vi "Teleop.vi"(0 "Call Context":T3) -> (1 "Loop 5 Value 1":dbl, 2 "Loop 5 Value 2":dbl, 3 "Loop 2 Value 2":dbl, 4 "Loop 2 Value 1":dbl, 6 "Loop 0 Value 1":dbl, 7 "Loop 1 Value 2":dbl, 8 "Loop 4 Value 2":dbl, 9 "SubState 5":T1, 10 "Loop 0 Value 2":dbl, 11 "Loop 1 Value 1":dbl, 12 "Loop 3 Value 2":dbl, 13 "Loop 3 Value 1":dbl, 14 "SubState 0":T2=enum."driver control", 15 "SubState 4":T2, 16 "SubState 3":T2, 17 "SubState 1":T2, 18 "Loop 4 Value 1":dbl, 19 "SubState 2":T2)   [LabVIEW 2011]
uses:
  subStates.ctl
  <vilib>/Rock Robotics/WPI/DriverStation/WPI_DriverStationDerivedRobotMode.ctl
  singleUseSubstate.ctl
  fg_typedef.ctl
  <vilib>/Rock Robotics/WPI/Solenoid/WPI_SolenoidValue.ctl
  <vilib>/Rock Robotics/WPI/Solenoid/WPI_SolenoidGetEnum.vi
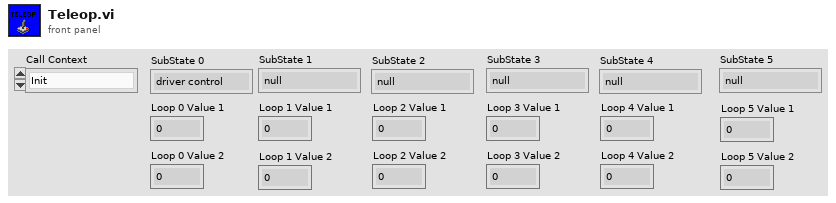
[diagram p1: front panel]
types:
  T1 = typedef "singleUseSubstate.ctl" = enum16{"null", "wait", "shift", "shift high", "shift low", "bridge down", "bridge up", "extender in", "extender out", "extender toggle", "end"}
  T2 = typedef "subStates.ctl" = enum16{"null", "wait", "driver control", "auto", "manual override", "autoDrive", "hold position", "rotate", "end"}
  T3 = typedef "WPI_DriverStationDerivedRobotMode.ctl" = enum16{"Init", "Execute", "Stop"}
  T4 = typedef "fg_typedef.ctl" = enum16{"Get", "Set"}
  T5 = typedef "WPI_JoystickDevRef.ctl" = cluster{"Device":T6}
  T6 = typedef "WPI_JoystickDeviceEnum.ctl" = enum16{"USB 1", "USB 2", "USB 3", "USB 4", "Kinect 1", "Kinect 2"}
  T7 = typedef "WPI_JoystickButtonState.ctl" = cluster{"Button 1":bool, "Button 2":bool, "Button 3":bool, "Button 4":bool, "Button 5":bool, "Button 6":bool, "Button 7":bool, "Button 8":bool, "Button 9":bool, "Button 10":bool, "Button 11":bool, "Button 12":bool}
  T8 = cluster{"axis 1 (x)":dbl, "axis 2 (y)":dbl, "axis 3 (throttle)":dbl, "axis 4":dbl, "axis 5":dbl, "axis 6":dbl}
  T9 = typedef "WPI_EncoderDevRef.ctl" = cluster{"DevStatus":errorcluster, "EncoderIndex":T10, "CounterIndex":T11, "DistancePerCount":dbl, "Decoding Type":T12}
  T10 = typedef "FPGA_EncoderIdx.ctl" = enum8{"Enc 0", "Enc 1", "Enc 2", "Enc 3", "Invalid"}
  T11 = typedef "FPGA_CounterCtrSystemIndex.ctl" = enum8{"Ctr 0", "Ctr 1", "Ctr 2", "Ctr 3", "Ctr 4", "Ctr 5", "Ctr 6", "Ctr 7", "Invalid"}
  T12 = typedef "WPI_EncoderType.ctl" = enum16{"1x", "2x", "4x"}
  T13 = typedef "WPI_SolenoidValue.ctl" = enum16{"Off", "On", "Forward", "Reverse"}
  T14 = typedef "WPI_SolenoidDevRef.ctl" = cluster{"DevStatus":errorcluster, "Solenoid Module":T15, "Forward Solenoid Channel":T16, "Reverse Solenoid Channel":T16}
  T15 = typedef "FPGA_TypedefSolenoidModule.ctl" = enum16{"Solenoid Module 1", "Solenoid Module 2"}
  T16 = typedef "WPI_SolenoidChannel.ctl" = enum8{"Solenoid 1", "Solenoid 2", "Solenoid 3", "Solenoid 4", "Solenoid 5", "Solenoid 6", "Solenoid 7", "Solenoid 8", "Invalid"}
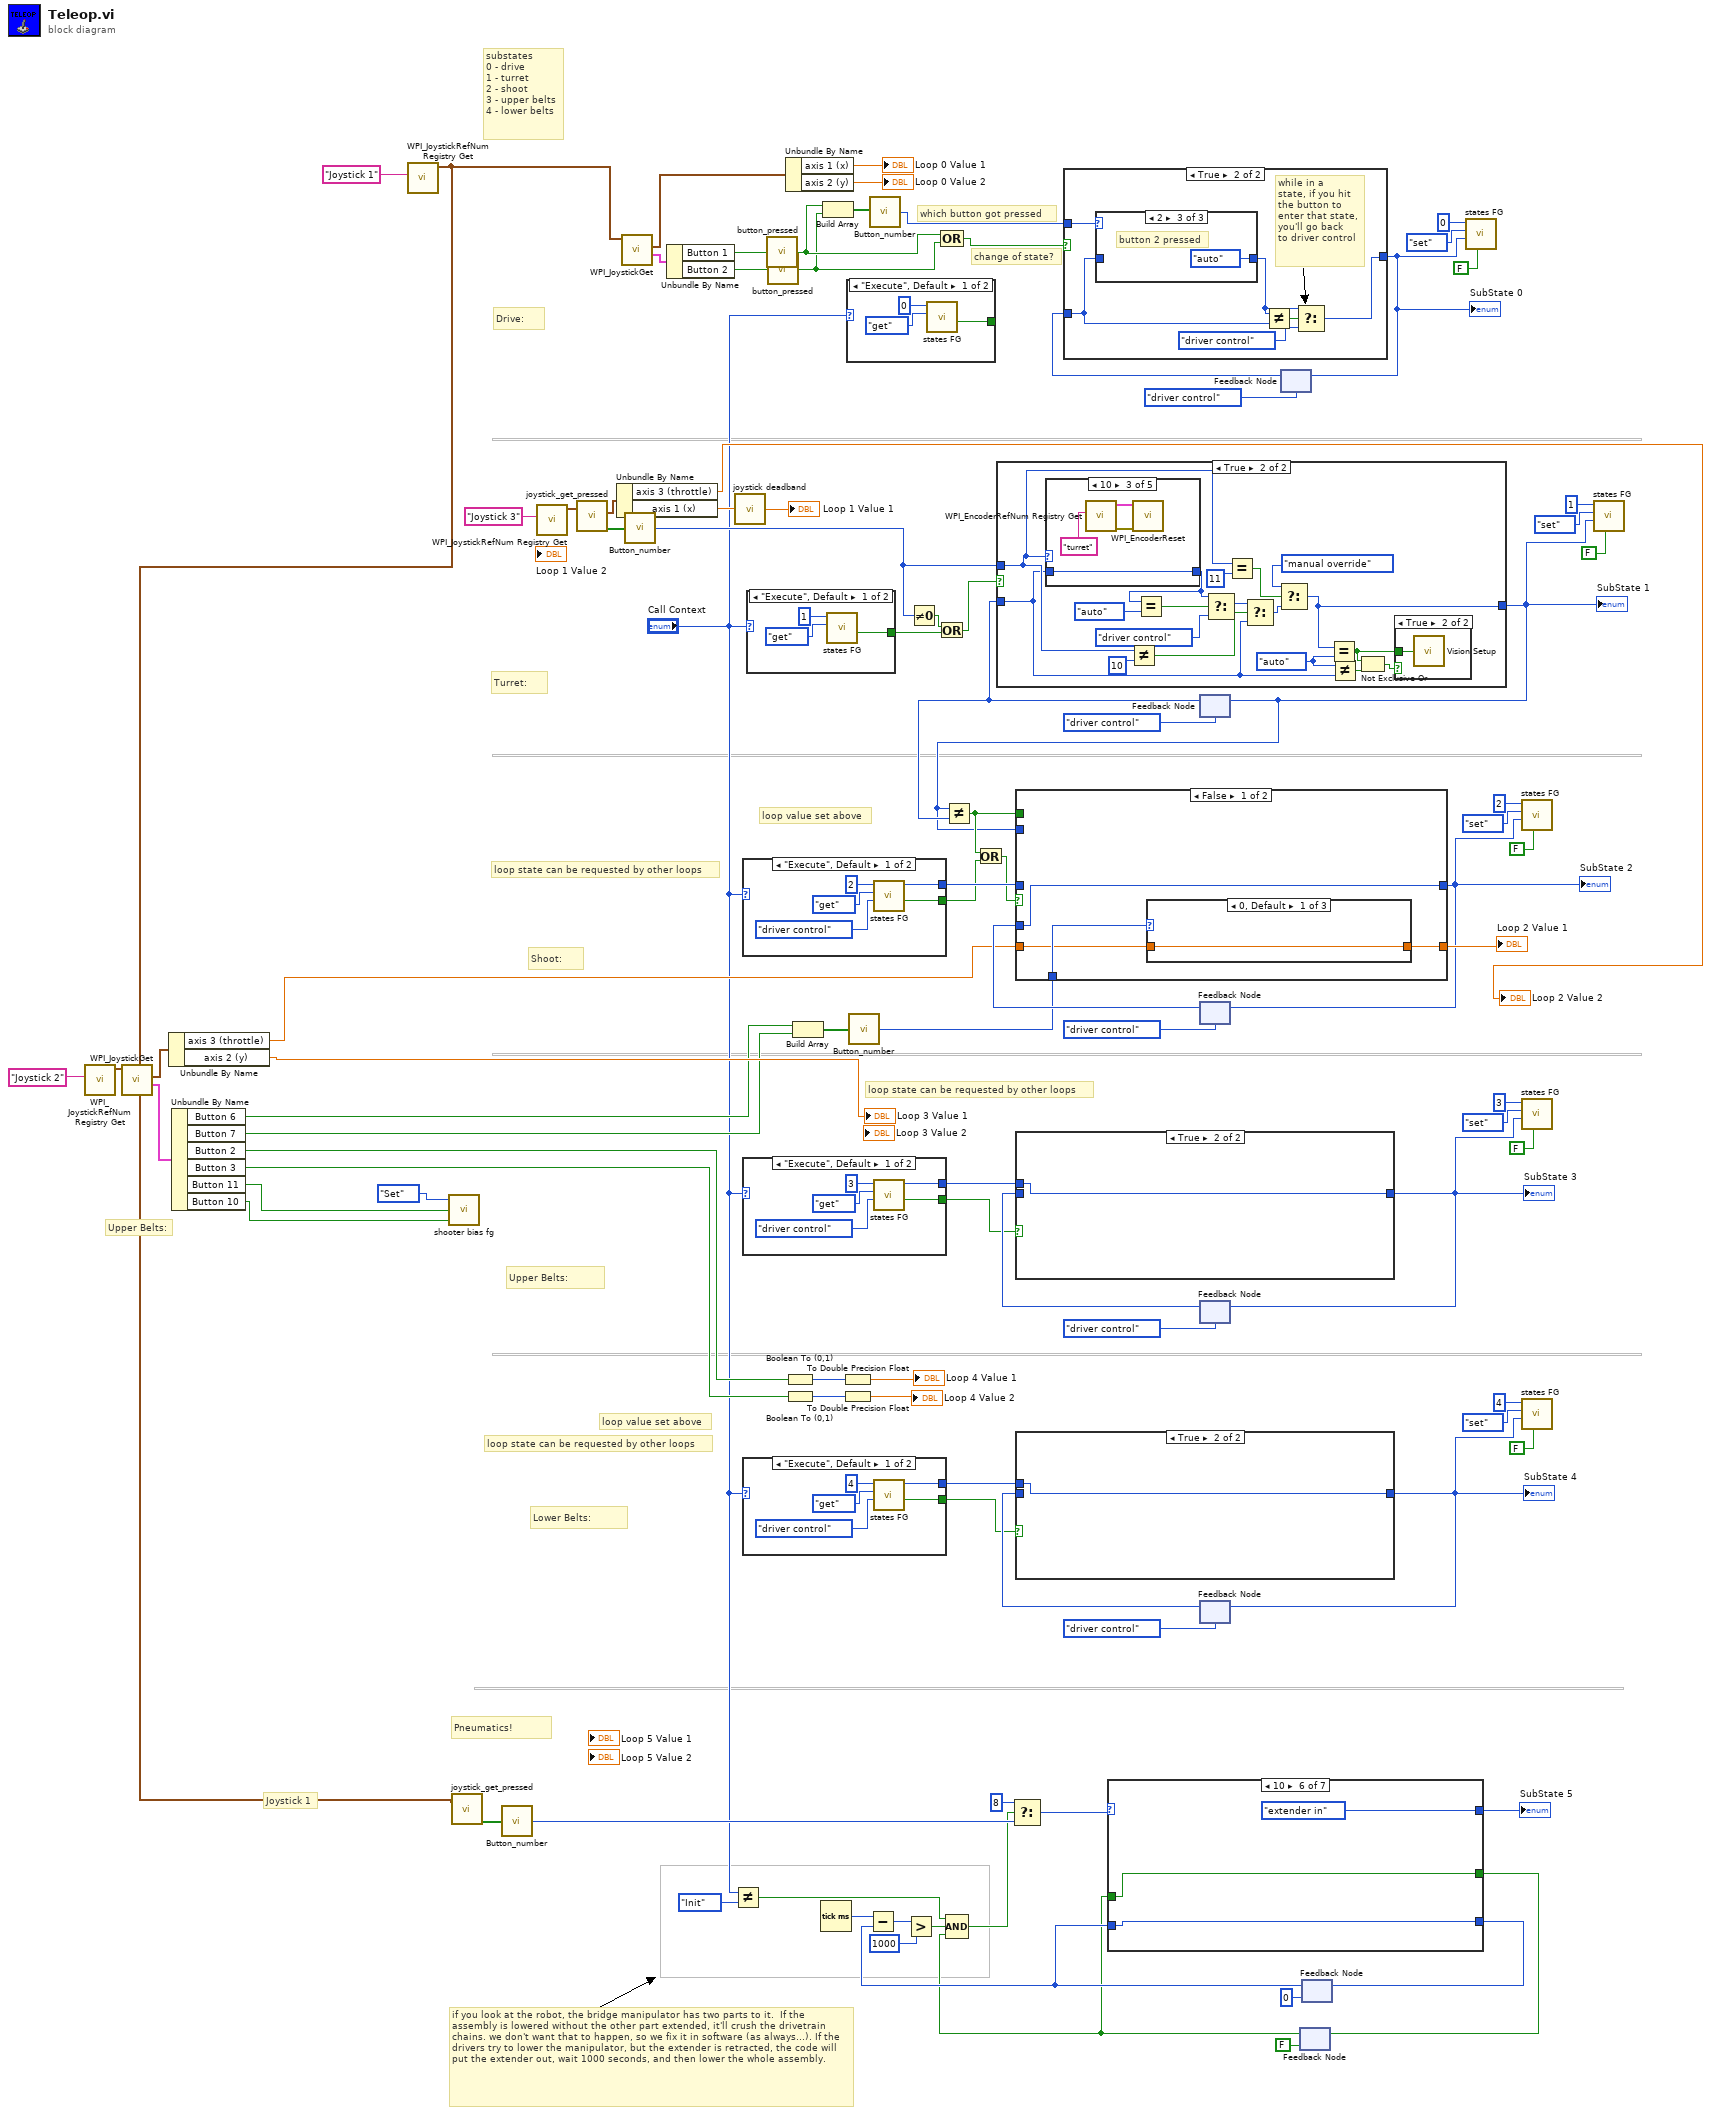
[diagram p0: block diagram]
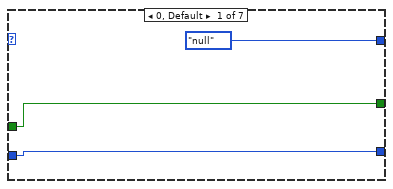
[diagram p2: hidden frame]
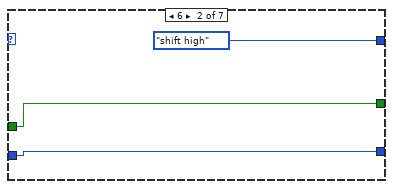
[diagram p3: hidden frame]
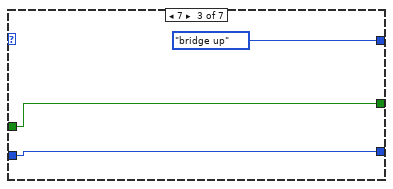
[diagram p4: hidden frame]
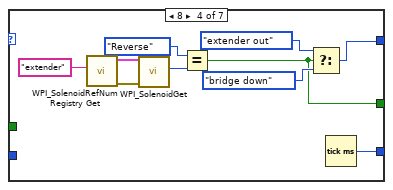
[diagram p5: hidden frame]
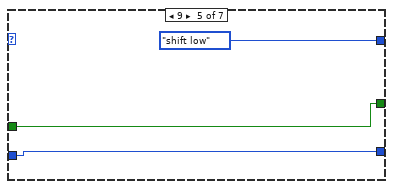
[diagram p6: hidden frame]
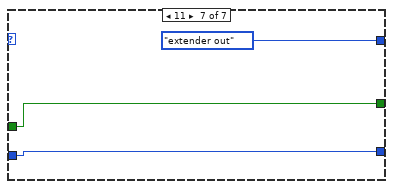
[diagram p7: hidden frame]
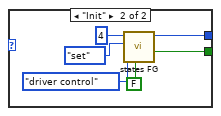
[diagram p9: hidden frame]
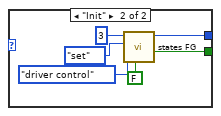
[diagram p11: hidden frame]
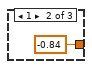
[diagram p12: hidden frame]
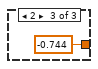
[diagram p13: hidden frame]
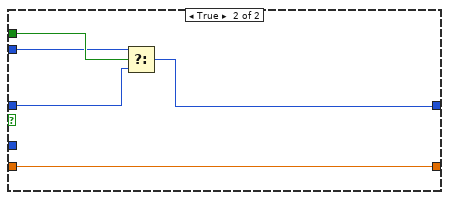
[diagram p14: hidden frame]
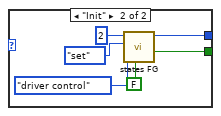
[diagram p15: hidden frame]
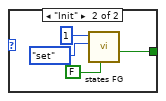
[diagram p16: hidden frame]
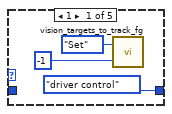
[diagram p19: hidden frame]
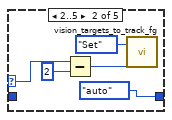
[diagram p20: hidden frame]
diagram:
  # "if you look at the robot, the bridge manipulator has two parts to it.  If the assembly is lowered without the other part extended, it'll crush the drivetrain chains. we don't want that to happen, so we fix it in software (as always...). If the drivers try to lower the manipulator, but the extender is retracted, the code will put the extender out, wait 1000 seconds, and then lower the whole assembly."
  # "change of state?"
  # "which button got pressed"
  # "Upper Belts:"
  # "Pneumatics!"
  # "Joystick 1"
  # "Lower Belts:"
  # "Upper Belts:"
  # "Shoot:"
  # "Turret:"
  # "Drive:"
  # "loop value set above"
  # "loop state can be requested by other loops"
  # "loop value set above"
  # "loop state can be requested by other loops"
  # "loop state can be requested by other loops"
  # "substates\n0 - drive\n1 - turret\n2 - shoot\n3 - upper belts\n4 - lower belts"
  n1 = call <vilib>:"WPI_JoystickRefNum Registry Get.vi"("refnum name"="Joystick 2") -> ("JoystickDevRef"=w57:T5)  [unwired: 9 in, 1 out]
  n2 = call <vilib>:"WPI_JoystickGet.vi"("JoystickDevRef"=w57) -> ("Buttons"=w55:T7, "Axes"=w56:T8)  [unwired: 4 in, 1 out]
  n3 = Unbundle By Name(w56) -> ("axis 3 (throttle)"=w30:dbl, "axis 2 (y)"=→"Loop 3 Value 1":dbl)
  n4 = Unbundle By Name(w55) -> ("Button 6"=w34:bool, "Button 7"=w33:bool, "Button 2"=w63:bool, "Button 3"=w62:bool, "Button 11"=w7:bool, "Button 10"=w6:bool)
  n5 = call <vilib>:"WPI_JoystickRefNum Registry Get.vi"("refnum name"="Joystick 1") -> ("JoystickDevRef"=w12:T5)  [unwired: 9 in, 1 out]
  n6 = call "shooter bias fg.vi"("Button 10 (dec)"=w6, "Button 11 (inc)"=w7, "Menu"=fg_typedef."Set") -> ()  [unwired: 1 out]
  n7 = call "joystick_get_pressed.vi"("JoystickDevRef 2"=w12) -> ("Buttons Pressed?"=w26:bool[])  [unwired: 1 in, 3 out]
  n8 = call "Button_number.vi"("Button Array"=w26) -> ("Button Pressed"=w15:i32)
  n9 = call <vilib>:"WPI_JoystickRefNum Registry Get.vi"("refnum name"="Joystick 3") -> ("JoystickDevRef"=w54:T5)  [unwired: 9 in, 1 out]
  n10 = call "joystick_get_pressed.vi"("JoystickDevRef 2"=w54) -> ("Axes"=w39:T8, "Buttons Pressed?"=w53:bool[])  [unwired: 1 in, 2 out]
  n11 = Unbundle By Name(w39) -> ("axis 3 (throttle)"=→"Loop 2 Value 2":dbl, "axis 1 (x)"=w28:dbl)
  n12 = call <vilib>:"WPI_JoystickGet.vi"("JoystickDevRef"=w12) -> ("Buttons"=w47:T7, "Axes"=w41:T8)  [unwired: 4 in, 1 out]
  n13 = call "Button_number.vi"("Button Array"=w53) -> ("Button Pressed"=w58:i32)
  n14 = Unbundle By Name(w47) -> ("Button 1"=w10:bool, "Button 2"=w35:bool)
  n15 = Not Equal?(x="Call Context", y=WPI_DriverStationDerivedRobotMode."Init") -> (x != y?=w3:bool)
  n16 = call "joystick deadband.vi"("Joystick In"=w28) -> ("Output"=→"Loop 1 Value 1":dbl)  [unwired: 4 in]
  n17 = case shown="\"Execute\", Default" "Call Context" {
    tunnel: [w104 w110] -> w51
    tunnel: [w102 w107] -> w52
    frame "Execute", Default {
      n18 = call "states FG.vi"("subState in"=subStates."driver control", "menu (get)"=enum16{"set", "get"}."get", "Loop ID"=2) -> ("exit out"=w104:bool, "subState out"=w102:T2)  [unwired: 5 in, 2 out]
    }
    frame "Init" {
      n19 = call "states FG.vi"("exit in"=FALSE, "subState in"=subStates."driver control", "menu (get)"=enum16{"set", "get"}."set", "Loop ID"=2) -> ("exit out"=w110:bool, "subState out"=w107:T2)  [unwired: 4 in, 2 out]
    }
  }
  n20 = case shown="\"Execute\", Default" "Call Context" {
    tunnel: [w115 w121] -> w68
    tunnel: [w114 w119] -> w83
    frame "Execute", Default {
      n21 = call "states FG.vi"("subState in"=subStates."driver control", "menu (get)"=enum16{"set", "get"}."get", "Loop ID"=3) -> ("exit out"=w115:bool, "subState out"=w114:T2)  [unwired: 5 in, 2 out]
    }
    frame "Init" {
      n22 = call "states FG.vi"("exit in"=FALSE, "subState in"=subStates."driver control", "menu (get)"=enum16{"set", "get"}."set", "Loop ID"=3) -> ("exit out"=w121:bool, "subState out"=w119:T2)  [unwired: 4 in, 2 out]
    }
  }
  n23 = case shown="\"Execute\", Default" "Call Context" {
    tunnel: [w126 w132] -> w61
    tunnel: [w125 w130] -> w69
    frame "Execute", Default {
      n24 = call "states FG.vi"("subState in"=subStates."driver control", "menu (get)"=enum16{"set", "get"}."get", "Loop ID"=4) -> ("exit out"=w126:bool, "subState out"=w125:T2)  [unwired: 5 in, 2 out]
    }
    frame "Init" {
      n25 = call "states FG.vi"("exit in"=FALSE, "subState in"=subStates."driver control", "menu (get)"=enum16{"set", "get"}."set", "Loop ID"=4) -> ("exit out"=w132:bool, "subState out"=w130:T2)  [unwired: 4 in, 2 out]
    }
  }
  n26 = case shown="\"Execute\", Default" "Call Context" {
    tunnel: [w135 w139] -> w60
    frame "Execute", Default {
      n27 = call "states FG.vi"("menu (get)"=enum16{"set", "get"}."get", "Loop ID"=1) -> ("exit out"=w135:bool)  [unwired: 6 in, 3 out]
    }
    frame "Init" {
      n28 = call "states FG.vi"("exit in"=FALSE, "menu (get)"=enum16{"set", "get"}."set", "Loop ID"=1) -> ("exit out"=w139:bool)  [unwired: 5 in, 3 out]
    }
  }
  n29 = call "button_pressed.vi"("Button In"=w10) -> ("Button Pressed?"=w45:bool)
  n30 = call "button_pressed.vi"("Button In"=w35) -> ("Button Pressed?"=w44:bool)
  n31 = Boolean To (0,1)(Boolean=w63) -> (0, 1=w66:i16)
  n32 = Boolean To (0,1)(Boolean=w62) -> (0, 1=w67:i16)
  n33 = Unbundle By Name(w41) -> ("axis 1 (x)"=→"Loop 0 Value 1":dbl, "axis 2 (y)"=→"Loop 0 Value 2":dbl)
  n34 = Build Array(w34, w33) -> (w32:bool[])
  n35 = Tick Count (ms)() -> (millisecond timer value=w21:u32)
  n36 = Build Array(w45, w44) -> (w43:bool[])
  n37 = To Double Precision Float(number=w66) -> (double precision float=→"Loop 4 Value 1":dbl)
  n38 = To Double Precision Float(number=w67) -> (double precision float=→"Loop 4 Value 2":dbl)
  n39 = case shown="\"Execute\", Default" "Call Context" {
    tunnel: [w142 w146] -> _
    frame "Execute", Default {
      n40 = call "states FG.vi"("menu (get)"=enum16{"set", "get"}."get", "Loop ID"=0) -> ("exit out"=w142:bool)  [unwired: 6 in, 3 out]
    }
    frame "Init" {
      n41 = call "states FG.vi"("exit in"=FALSE, "menu (get)"=enum16{"set", "get"}."set", "Loop ID"=0) -> ("exit out"=w146:bool)  [unwired: 5 in, 3 out]
    }
  }
  n42 = call "Button_number.vi"("Button Array"=w32) -> ("Button Pressed"=w31:i32)
  n43 = call "Button_number.vi"("Button Array"=w43) -> ("Button Pressed"=w42:i32)
  n44 = Not Equal To 0?(x=w58) -> (x != 0?=w59:bool)
  n45 = Or(x=w59, y=w60) -> (x .or. y?=w94:bool)
  n46 = Compound Arithmetic op=OR(w45, w44) -> (w46:bool)
  n47 = feedback #1(subStates."driver control" ("Drive SubState")) -> (w48:T2)
  n48 = case shown="True" w94 {
    tunnel: w48 -> [w149 w152]
    tunnel: [w149 w157] -> w40
    tunnel: w58 -> [_ w154]
    frame False {
    }
    frame True {
      w167 = subStates."auto" ("y")
      n49 = case shown="10" w154 {
        selector: w154 -> [_ w172 _ _ _]
        tunnel: [subStates."driver control" ("Drive SubState") subStates."auto" ("Drive SubState") w180 subStates."manual override" ("Drive SubState") w184] -> w162
        tunnel: w152 -> [_ _ w180 _ w184]
        frame 1 {
          n50 = call "vision_targets_to_track_fg.vi"("Input"=-1, "Menu (Get)"=fg_typedef."Set") -> ()  [unwired: 1 out]
        }
        frame 2..5 {
          n51 = Subtract(x=w172, y=2) -> (x-y=w173:i32)
          n52 = call "vision_targets_to_track_fg.vi"("Input"=w173, "Menu (Get)"=fg_typedef."Set") -> ()  [unwired: 1 out]
        }
        frame 10 {
          n53 = call <vilib>:"WPI_EncoderRefNum Registry Get.vi"("refnum name"="turret") -> ("error out"=w178:errorcluster, "EncoderDevRef"=w177:T9)  [unwired: 9 in]
          n54 = call <vilib>:"WPI_EncoderReset.vi"("error in (no error)"=w178, "EncoderDevRef"=w177) -> ()  [unwired: 8 in, 2 out]
        }
        frame 11 {
          n55 = call "vision_targets_to_track_fg.vi"("Input"=-1, "Menu (Get)"=fg_typedef."Set") -> ()  [unwired: 1 out]
        }
        frame Default {
        }
      }
      n56 = Not Equal?(x=w154, y=10) -> (x != y?=w153:bool)
      n57 = Equal?(x=w162, y=subStates."auto") -> (x = y?=w156:bool)
      n58 = Select(t=w162, s=w156, f=subStates."driver control" ("Drive SubState")) -> (s? t:f=w151:T2)
      n59 = Equal?(x=w154, y=11) -> (x = y?=w160:bool)
      n60 = Select(t=w151, s=w153, f=w152) -> (s? t:f=w150:T2)
      n61 = Select(t=subStates."manual override", s=w160, f=w150) -> (s? t:f=w157:T2)
      n62 = Equal?(x=w157, y=w167) -> (x = y?=w164:bool)
      n63 = Not Equal?(x=w167, y=w152) -> (x != y?=w166:bool)
      n64 = Not Exclusive Or(1:w166, 2:w164) -> (0:w165:bool)
      n65 = case shown="True" w165 {
        tunnel: w164 -> [_ w168]
        frame False {
        }
        frame True {
          n66 = call "Vision Setup.vi"("enable/disable"=w168) -> ()
        }
      }
    }
  }
  "SubState 1" <- w40
  n67 = Not Equal?(x=w40, y=w48) -> (x != y?=w49:bool)
  n68 = Or(x=w49, y=w51) -> (x .or. y?=w50:bool)
  n69 = feedback-in #1(w40) -> ()
  n70 = feedback #2(subStates."driver control" ("Drive SubState")) -> (w87:T2)
  n71 = case shown="False" w50 {
    tunnel: w87 -> [w188 _]
    tunnel: [w188 w193] -> w9
    tunnel: w52 -> [_ w194]
    tunnel: w49 -> [_ w196]
    tunnel: w40 -> [_ w195]
    tunnel: w31 -> [w187 _]
    tunnel: w30 -> [w186 w192]
    tunnel: [w185 w192] -> w29
    frame False {
      n72 = case shown="0, Default" w187 {
        tunnel: w186 -> [w189 _ _]
        tunnel: [w189 -0.84 ("axis 3 (throttle)") -0.744 ("axis 3 (throttle)")] -> w185
        frame 0, Default {
        }
        frame 1 {
        }
        frame 2 {
        }
      }
    }
    frame True {
      n73 = Select(t=w195, s=w196, f=w194) -> (s? t:f=w193:T2)
    }
  }
  "SubState 2" <- w9
  "Loop 2 Value 1" <- w29
  n74 = feedback-in #2(w9) -> ()
  n75 = feedback #3(subStates."driver control" ("Drive SubState")) -> (w78:T2)
  n76 = case shown="True" w68 {
    tunnel: w78 -> [w197 _]
    tunnel: [w197 w198] -> w82
    tunnel: w83 -> [_ w198]
    frame False {
    }
    frame True {
    }
  }
  "SubState 3" <- w82
  n77 = feedback-in #3(w82) -> ()
  n78 = feedback #4(subStates."driver control" ("Drive SubState")) -> (w74:T2)
  n79 = case shown="True" w61 {
    tunnel: w74 -> [w199 _]
    tunnel: [w199 w200] -> w70
    tunnel: w69 -> [_ w200]
    frame False {
    }
    frame True {
    }
  }
  "SubState 4" <- w70
  n80 = feedback-in #4(w70) -> ()
  n81 = feedback #5(subStates."driver control" ("Drive SubState")) -> (w89:T2)
  n82 = case shown="True" w46 {
    tunnel: w89 -> [w201 w205]
    tunnel: [w201 w206] -> w96
    tunnel: w42 -> [_ w202]
    frame False {
      # "keep current state, no change necessary"
    }
    frame True {
      # "while in a \nstate, if you hit\nthe button to\nenter that state,\nyou'll go back \nto driver control"
      n83 = case shown="2" w202 {
        tunnel: [w208 subStates."hold position" ("Drive SubState") subStates."auto" ("Drive SubState")] -> w203
        tunnel: w205 -> [w208 _ _]
        frame 0, Default {
          # "no button pressed"
        }
        frame 1 {
          # "button 1 pressed"
        }
        frame 2 {
          # "button 2 pressed"
        }
      }
      n84 = Not Equal?(x=w203, y=w205) -> (x != y?=w207:bool)
      n85 = Select(t=w203, s=w207, f=subStates."driver control") -> (s? t:f=w206:T2)
    }
  }
  "SubState 0" <- w96
  n86 = feedback-in #5(w96) -> ()
  n87 = feedback #6(FALSE) -> (w16:bool)
  n88 = feedback #7(u32 0 ("millisecond timer value")) -> (w20:u32)
  n89 = Subtract(x=w21, y=w20) -> (x-y=w19:u32)
  n90 = Greater?(x=w19, y=u32 1000) -> (0:w17:bool)
  n91 = Compound Arithmetic op=AND(w3, w17, w16) -> (w5:bool)
  n92 = Select(t=8, s=w5, f=w15) -> (s? t:f=w14:i32)
  n93 = case shown="10" w14 {
    tunnel: [singleUseSubstate."null" ("Enum") singleUseSubstate."shift high" ("Enum") singleUseSubstate."bridge up" ("Enum") w222 singleUseSubstate."shift low" ("Enum") singleUseSubstate."extender in" ("Enum") singleUseSubstate."extender out" ("Enum")] -> w4
    tunnel: [w212 w215 w218 w221 w231 w234 w237] -> w25
    tunnel: w20 -> [w212 w215 w218 _ w231 w234 w237]
    tunnel: [w211 w214 w217 w220 w230 w233 w236] -> w23
    tunnel: w16 -> [w211 w214 w217 _ w230 w233 w236]
    frame 0, Default {
    }
    frame 6 {
    }
    frame 7 {
    }
    frame 8 {
      n94 = call <vilib>:"WPI_SolenoidRefNum Registry Get.vi"("refnum name"="extender") -> ("error out"=w228:errorcluster, "SolenoidDevRef"=w227:T14)  [unwired: 9 in]
      n95 = call-poly <vilib>:"WPI_SolenoidGet.vi"("error in (no error)"=w228, "SolenoidDevRef"=w227) -> ("Value"=w226:T13)  [unwired: 7 in, 2 out]
      n96 = Equal?(x=WPI_SolenoidValue."Reverse", y=w226) -> (x = y?=w220:bool)
      n97 = Select(t=singleUseSubstate."extender out" ("Enum"), s=w220, f=singleUseSubstate."bridge down") -> (s? t:f=w222:T1)
      n98 = Tick Count (ms)() -> (millisecond timer value=w221:u32)
    }
    frame 9 {
    }
    frame 10 {
    }
    frame 11 {
    }
  }
  "SubState 5" <- w4
  n99 = feedback-in #6(w23) -> ()
  n100 = feedback-in #7(w25) -> ()
  n101 = call "states FG.vi"("exit in"=FALSE, "subState in"=w96, "menu (get)"=enum16{"set", "get"}."set", "Loop ID"=0) -> ()  [unwired: 4 in, 4 out]
  n102 = call "states FG.vi"("exit in"=FALSE, "subState in"=w9, "menu (get)"=enum16{"set", "get"}."set", "Loop ID"=2) -> ()  [unwired: 4 in, 4 out]
  n103 = call "states FG.vi"("exit in"=FALSE, "subState in"=w82, "menu (get)"=enum16{"set", "get"}."set", "Loop ID"=3) -> ()  [unwired: 4 in, 4 out]
  n104 = call "states FG.vi"("exit in"=FALSE, "subState in"=w70, "menu (get)"=enum16{"set", "get"}."set", "Loop ID"=4) -> ()  [unwired: 4 in, 4 out]
  n105 = call "states FG.vi"("exit in"=FALSE, "subState in"=w40, "menu (get)"=enum16{"set", "get"}."set", "Loop ID"=1) -> ()  [unwired: 4 in, 4 out]
